vi "_Get or Add Workbookpart.vi"(8 "error in":errorcluster, 11 "SpreadsheetDocument":refnum<k24>) -> (0 "error out":errorcluster, 2 "WorkbookPart":refnum<k24>, 3 "SpreadsheetDocument out":refnum<k24>)   [LabVIEW 2021, in "Open Xml.lvlib"]
uses:
  Open Xml.lvlib
  D:/git/Open-Xml-LabVIEW/dll/DocumentFormat.OpenXml.dll
  dll/DocumentFormat.OpenXml.dll
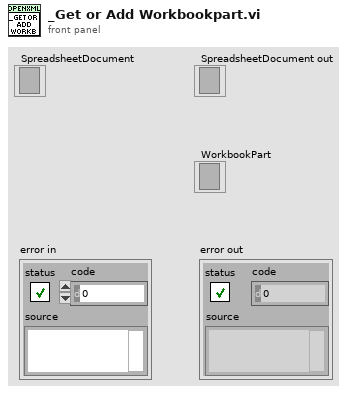
[diagram p1: front panel]
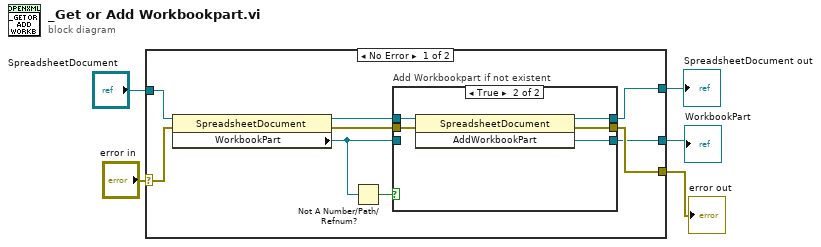
[diagram p0: block diagram]
diagram:
  n1 = case shown="No Error" "error in" {
    selector: "error in" -> [w14 w23]
    tunnel: [w7 w23] -> w4
    tunnel: "SpreadsheetDocument" -> [w13 _]
    tunnel: [w8 _] -> w2
    tunnel: [w6 _] -> w1
    frame No Error {
      n2 = property class="SpreadsheetDocument"(reference=w13, error in=w14) -> (reference out=w10:refnum<k24>, error out=w9:errorcluster, "WorkbookPart"=w11:refnum<k24>)
      n3 = Not A Number/Path/Refnum?(number/path/refnum=w11) -> (NaN/Path/Refnum?=w12:bool)
      n4 = case "Add Workbookpart if not existent" shown="True" w12 {
        tunnel: w11 -> [w15 _]
        tunnel: w10 -> [w16 w22]
        tunnel: w9 -> [w17 w21]
        tunnel: [w16 w20] -> w8
        tunnel: [w17 w19] -> w7
        tunnel: [w15 w18] -> w6
        frame False {
        }
        frame True {
          n5 = invoke class="SpreadsheetDocument" method="AddWorkbookPart"(reference=w22, error in=w21) -> (reference out=w20:refnum<k24>, error out=w19:errorcluster, "AddWorkbookPart"=w18:refnum<k24>)  [unwired: 1 in]
        }
      }
    }
    frame Error {
    }
  }
  "error out" <- w4
  "SpreadsheetDocument out" <- w2
  "WorkbookPart" <- w1
